vi "Error Check.vi"(11 "Input":string) -> (3 "Error":bool)   [LabVIEW 2017]
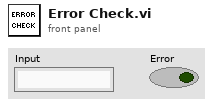
[diagram p1: front panel]
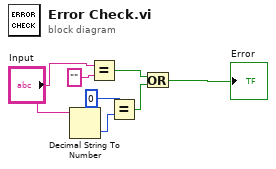
[diagram p0: block diagram]
diagram:
  n1 = Decimal String To Number(string="Input") -> (number=w7:i32)  [unwired: 2 in, 1 out]
  n2 = Equal?(x="Input", y="") -> (x = y?=w5:bool)
  n3 = Equal?(x=0, y=w7) -> (x = y?=w4:bool)
  n4 = Or(x=w5, y=w4) -> (x .or. y?=→"Error":bool)
